vi "Autonomous Independent.vi"() -> ()   [LabVIEW 2015]
doc: "This VI is called when autonomous begins, and will automatically be terminated when autonomous ends. You can carry out timed or sensor driven robot movement independently without needing to return to the caller."
uses:
  Auto States.ctl
  <vilib>/Rock Robotics/WPI/Utilities/WPI_GetSetVariantRefNum.vi
  <vilib>/Rock Robotics/Network Tables/NT Write Numeric Array.vi
  <vilib>/Rock Robotics/Network Tables/NT Read Boolean.vi
  Robot Global Data.vi
  <vilib>/Rock Robotics/Network Tables/NT Read String.vi
  Sensors.vi
panel:
  out "x >= y?":bool
  out "Enum":T1
  out "Complete":bool=TRUE
  out "Crossed":bool
  # "Be sure to right-click and choose Data Operations>>Make Current Value default if you want to save the array values with the VI"
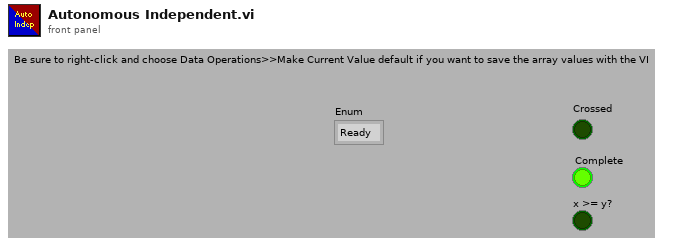
[diagram p1: front panel]
types:
  T1 = typedef "Auto States.ctl" = enum16{"Ready", "Drive to Obstacle", "Cross the Obstacle", "Pause before proceeding", "Position robot for shooting", "Complete"}
  T2 = typedef "WPI_JoystickDevRef.ctl" = cluster{"Device":T3}
  T3 = typedef "WPI_JoystickDeviceEnum.ctl" = enum16{"USB 0", "USB 1", "USB 2", "USB 3", "USB 4", "USB 5"}
  T4 = cluster{"Rotational Value":dbl, "Translational  Value":dbl}
  T5 = typedef "WPI_DigitalInputDevRef.ctl" = cluster{"DevStatus":errorcluster, "DIO Channel":T6}
  T6 = typedef "FPGA_DIOChannel.ctl" = enum8{"DIO 0", "DIO 1", "DIO 2", "DIO 3", "DIO 4", "DIO 5", "DIO 6", "DIO 7", "DIO 8", "DIO 9", "DIO MXP 0", "DIO MXP 1", "DIO MXP 2", "DIO MXP 3", "DIO MXP 4", "DIO MXP 5", "DIO MXP 6", "DIO MXP 7", "DIO MXP 8", "DIO MXP 9", "DIO MXP 10", "DIO MXP 11", "DIO MXP 12", "DIO MXP 13", "DIO MXP 14", "DIO MXP 15", "Invalid"}
  T7 = cluster{"Translational speed":dbl, "Rotational speed":dbl}
  T8 = cluster{"Rotational Velocity Deployed":dbl, "Translational Velocity Deployed":dbl}
  T9 = typedef "WPI_MotorControlDeviceRef.ctl" = cluster{"DeviceStatus":errorcluster, "Type":T10, "PWM":cluster{"PWM Channel":T11, "DeadBand":T12}, "CAN":cluster{"Device Number":u8, "Control Mode":T13, "Semaphore":T14, "Max Vout":dbl, "TalonSRX Control Mode":T15}, "Invert":bool}
  T10 = typedef "WPI_MotorControlType.ctl" = enum16{"PWM", "CAN", "CANTalonSRX"}
  T11 = typedef "FPGA_DIOPWMChannel.ctl" = enum8{"PWM 0", "PWM 1", "PWM 2", "PWM 3", "PWM 4", "PWM 5", "PWM 6", "PWM 7", "PWM 8", "PWM 9", "PWM MXP 0", "PWM MXP 1", "PWM MXP 2", "PWM MXP 3", "PWM MXP 4", "PWM MXP 5", "PWM MXP 6", "PWM MXP 7", "PWM MXP 8", "PWM MXP 9", "Invalid"}
  T12 = typedef "WPI_PWMDeadband.ctl" = cluster{"Name":string, "maxPositivePwm":i32, "minPositivePwm":i32, "centerPwm":i32, "maxNegativePwm":i32, "minNegativePwm":i32, "angularRange":u16}
  T13 = typedef "WPI_CANJaguar_ControlMode.ctl" = enum8{"Percent VBus", "Current", "Speed", "Position", "Voltage"}
  T14 = typedef "Semaphore RefNum" = refnum<k1>
  T15 = typedef "WPI_CANTalonSRX_APIControlMode.ctl" = enum8{"Percent VBus", "Speed", "Position", "Slave", "Unchanged / Invalid", "Voltage Compensation", "Current", "Motion Profile"}
  T16 = typedef "WPI_RobotDriveDevRef.ctl" = cluster{"DevStatus":errorcluster, "Motors[]":T9[], "Square Inputs":bool, "Max Output":dbl}
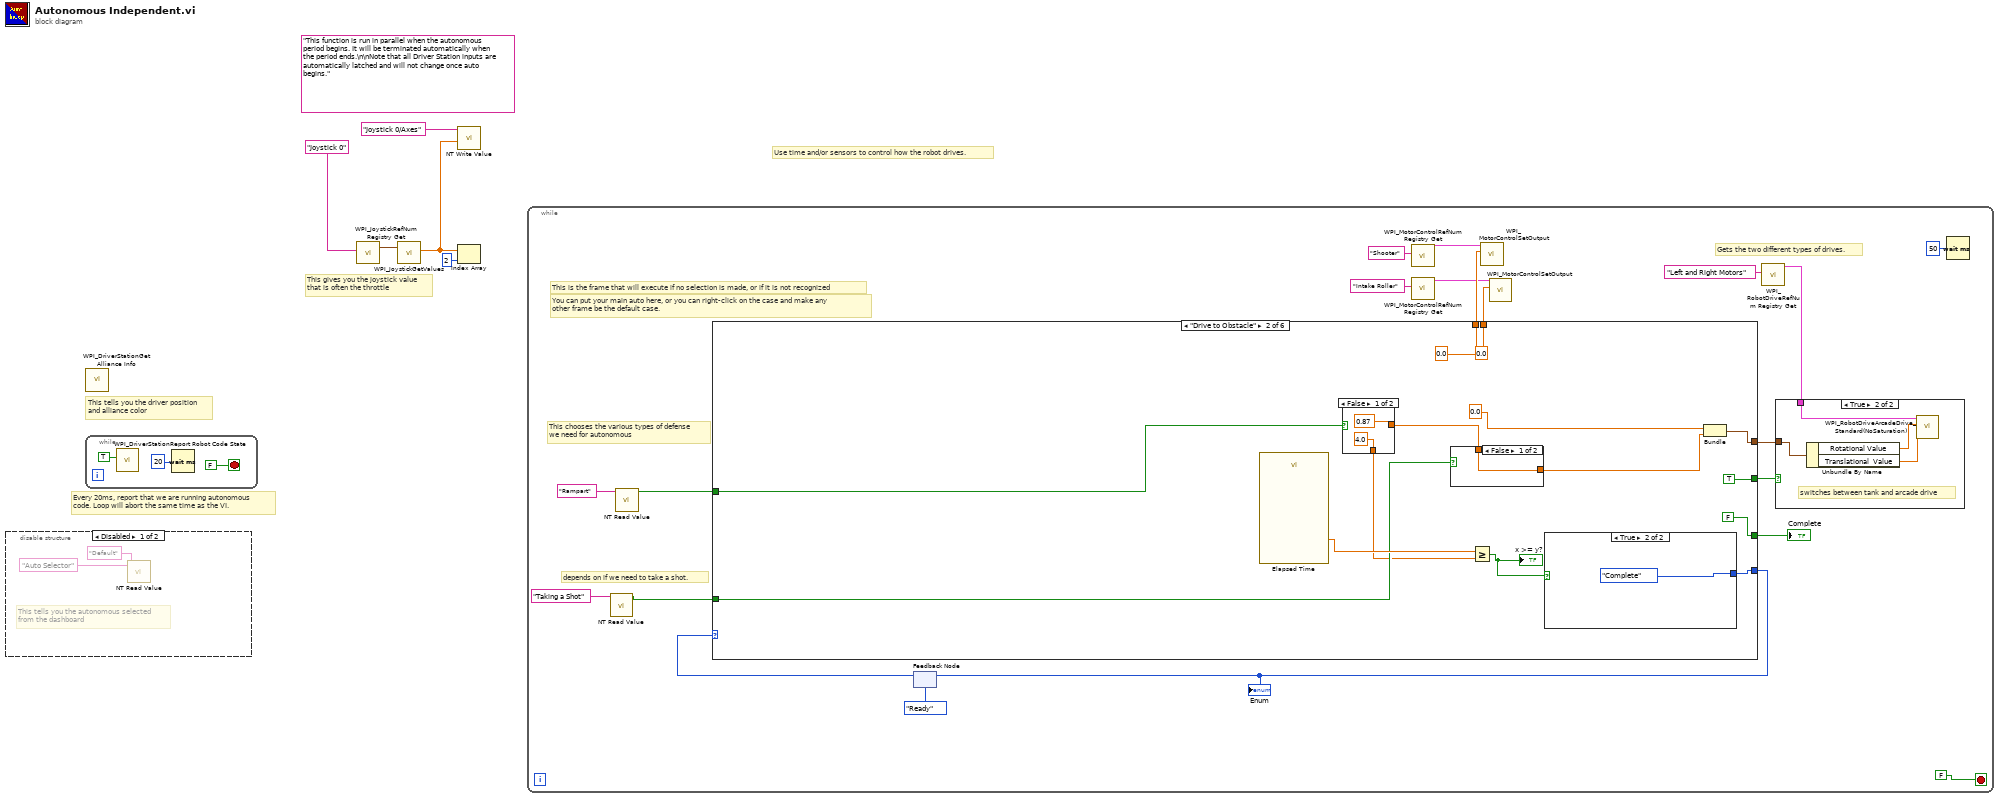
[diagram p0: block diagram]
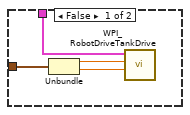
[diagram p2: hidden frame]
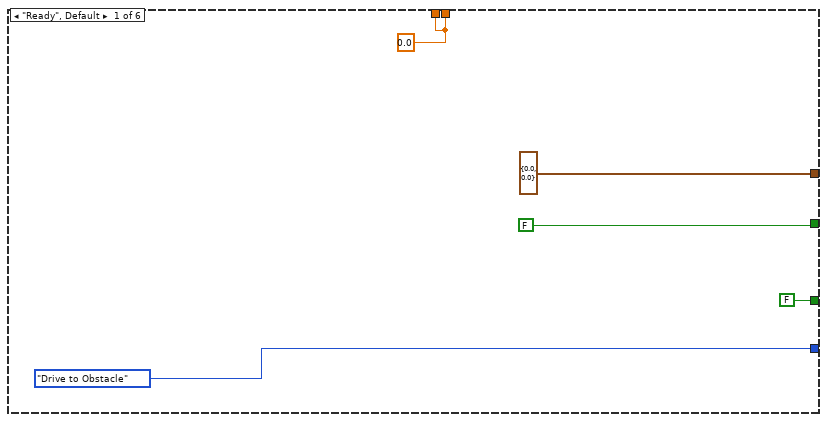
[diagram p3: hidden frame]
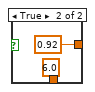
[diagram p4: hidden frame]
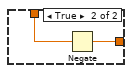
[diagram p5: hidden frame]
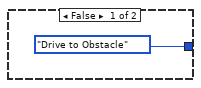
[diagram p6: hidden frame]
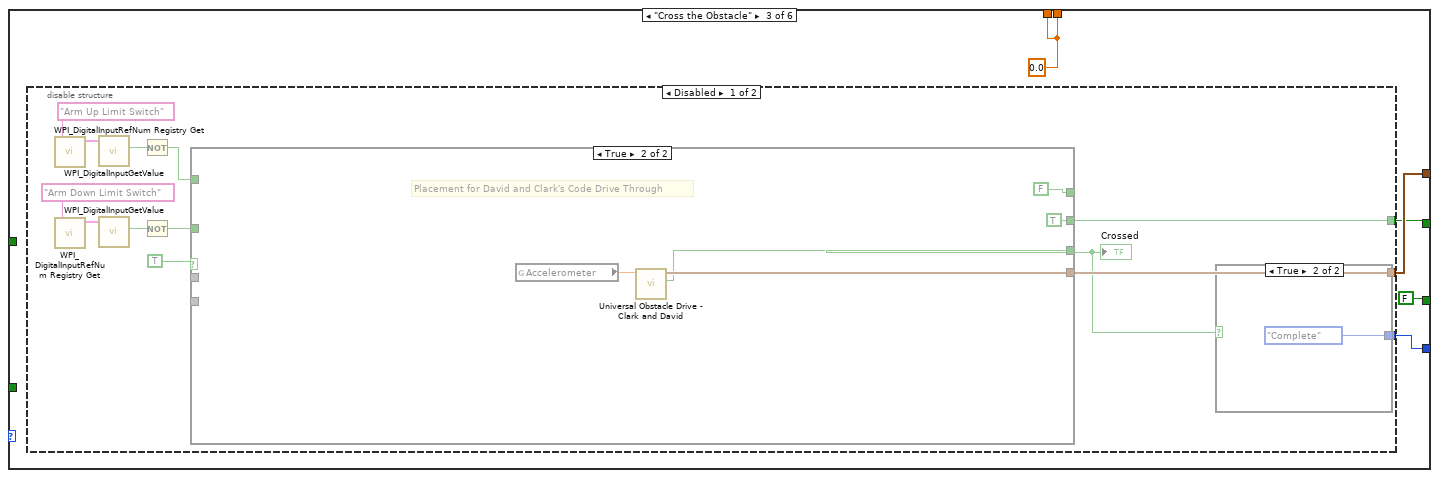
[diagram p7: hidden frame]
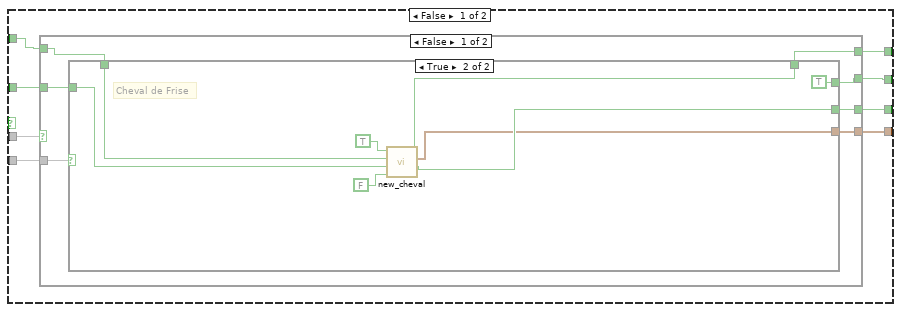
[diagram p8: hidden frame]
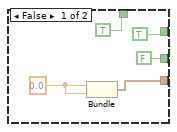
[diagram p9: hidden frame]
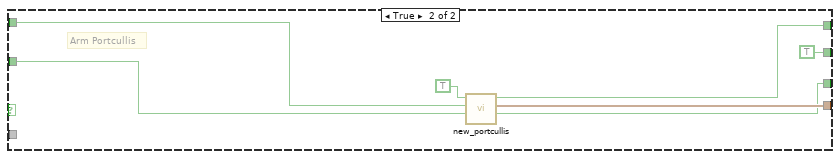
[diagram p10: hidden frame]
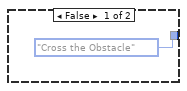
[diagram p11: hidden frame]
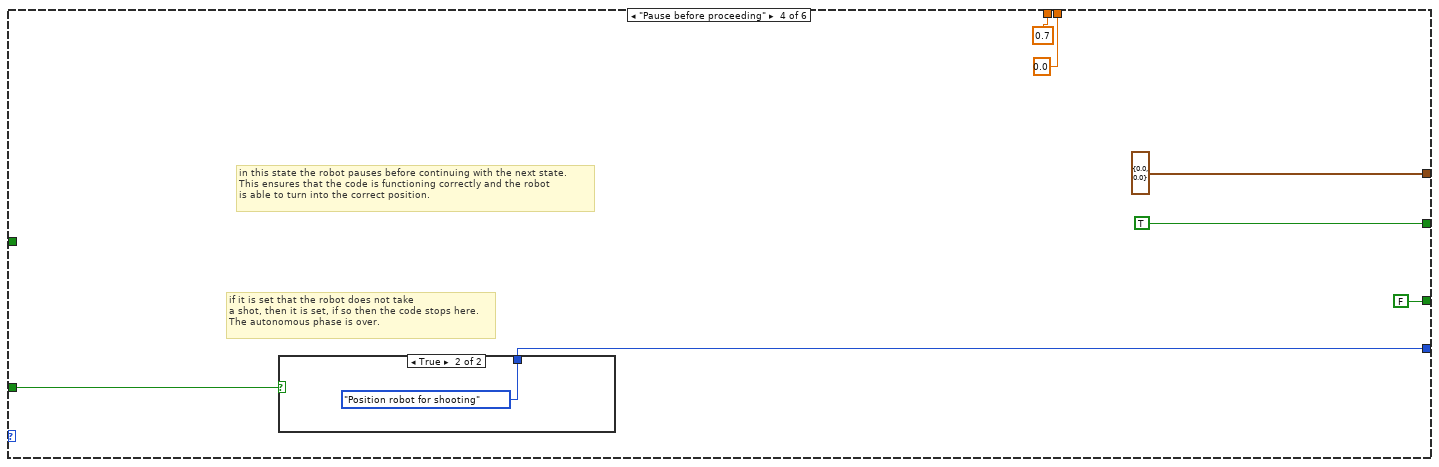
[diagram p13: hidden frame]
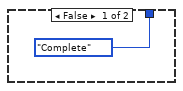
[diagram p14: hidden frame]
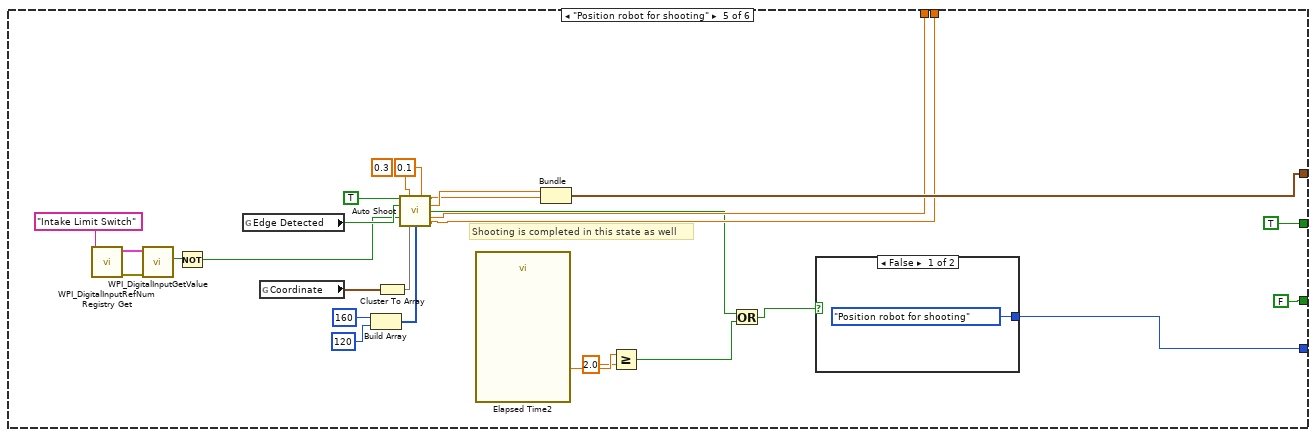
[diagram p15: hidden frame]
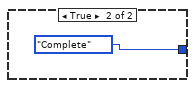
[diagram p16: hidden frame]
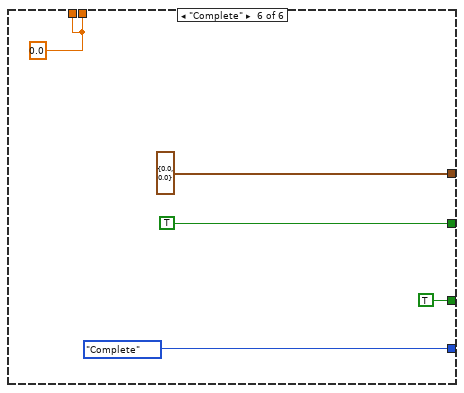
[diagram p17: hidden frame]
diagram:
  (unwired) "This function is run in parallel when the autonomous period begins. It will be terminated automatically when the period ends.\n\nNote that all Driver Station inputs are automatically latched and will not change once auto begins."
  # "Every 20ms, report that we are running autonomous\ncode. Loop will abort the same time as the VI."
  # "This gives you the joystick value\nthat is often the throttle"
  # "Use time and/or sensors to control how the robot drives."
  # "This tells you the driver position\nand alliance color"
  n1 = disable-structure shown="Disabled" {
    frame Disabled {
      # "This tells you the autonomous selected\nfrom the dashboard"
      n2 = call-poly <vilib>:"NT Read Value.vi"("Default Value"="Default", "Name"="Auto Selector") -> ("String"=w7:string)  [unwired: 8 in, 1 out]
    }
    frame Enabled {
    }
  }
  n3 = while {
    stop <- FALSE stop-if-true
    n4 = call <vilib>:"WPI_DriverStationReport Robot Code State.vi"("Autonomous"=TRUE) -> ()  [unwired: 10 in, 1 out]
    n5 = Wait (ms)(milliseconds to wait=u32 20) -> ()  [unwired: 1 out]
  }
  n6 = call <vilib>:"WPI_DriverStationGet Alliance Info.vi"() -> ()  [unwired: 12 out]
  n7 = call <vilib>:"WPI_JoystickRefNum Registry Get.vi"("refnum name"="Joystick 0") -> ("JoystickDevRef"=w4:T2)  [unwired: 1 in, 9 out]
  n8 = call <vilib>:"WPI_JoystickGetValues.vi"("JoystickDevRef"=w4) -> ("Axes"=w2:dbl[])  [unwired: 6 in, 4 out]
  n9 = call-poly <vilib>:"NT Write Value.vi"("Numeric Array"=w2, "Name"="Joystick 0/Axes") -> ()  [unwired: 9 in, 1 out]
  n10 = Index Array(array=w2, index=2) -> ()  [unwired: 1 out]
  n11 = while {
    stop <- FALSE stop-if-true
    # "depends on if we need to take a shot."
    # "Gets the two different types of drives."
    # "This chooses the various types of defense\nwe need for autonomous"
    # "You can put your main auto here, or you can right-click on the case and make any\nother frame be the default case."
    # "This is the frame that will execute if no selection is made, or if it is not recognized"
    n12 = call-poly <vilib>:"NT Read Value.vi"("Name"="Taking a Shot") -> ("Boolean"=w15:bool)  [unwired: 9 in, 1 out]
    n13 = call-poly <vilib>:"NT Read Value.vi"("Name"="Rampart") -> ("Boolean"=w12:bool)  [unwired: 9 in, 1 out]
    n14 = feedback #1(Auto_States."Ready") -> (w23:T1)
    n15 = case shown="\"Drive to Obstacle\"" w23 {
      tunnel: [Auto_States."Drive to Obstacle" w55 w71 w133 w162 Auto_States."Complete"] -> w22
      tunnel: [FALSE TRUE w70 TRUE ("Arcada Drive?") TRUE TRUE ("Arcada Drive?")] -> w30
      tunnel: [T4 {"Rotational Value"=0.0, "Translational  Value"=0.0} ("Aracade Drive") w57 w72 T4 {"Rotational Value"=0.0, "Translational  Value"=0.0} ("Aracade Drive") w159 T4 {"Rotational Value"=0.0, "Translational  Value"=0.0} ("Aracade Drive")] -> w29
      tunnel: w15 -> [_ w49 _ w134 _ _]
      tunnel: [FALSE FALSE FALSE FALSE FALSE TRUE] -> w27
      tunnel: [w40 0.0 w68 0.7 ("Shooter") w151 w165] -> w19
      tunnel: [w40 0.0 w68 0.0 w150 w165] -> w17
      tunnel: w12 -> [_ w45 _ _ _ _]
      frame "Ready", Default {
        w40 = 0.0
      }
      frame "Drive to Obstacle" {
        n16 = call "Elapsed Time"() -> ("Elapsed Time (s)"=w54:dbl)  [unwired: 12 in, 7 out]
        n17 = case shown="False" w45 {
          tunnel: [0.87 0.92 ("Desired Angle")] -> w48
          tunnel: [4.0 6.0 ("y")] -> w46
          frame False {
          }
          frame True {
          }
        }
        n18 = case shown="False" w49 {
          tunnel: w48 -> [w63 w65]
          tunnel: [w63 w64] -> w47
          frame False {
          }
          frame True {
            n19 = Negate(x=w65) -> (-x=w64:dbl)
          }
        }
        n20 = Greater Or Equal?(x=w54, y=w46) -> (x >= y?=w50:bool)
        "x >= y?" <- w50
        n21 = case shown="True" w50 {
          tunnel: [Auto_States."Drive to Obstacle" Auto_States."Complete"] -> w55
          frame False {
          }
          frame True {
          }
        }
        n22 = Bundle("Speed"=0.0, "Desired Angle"=w47) -> (w57:cluster{"Speed":dbl, "Desired Angle":dbl})  [unwired: 1 in]
      }
      frame "Cross the Obstacle" {
        w68 = 0.0
        n23 = disable-structure shown="Disabled" {
          disable-tunnel: [w85 _] -> w72
          disable-tunnel: [w83 _] -> w71
          disable-tunnel: [w82 _] -> w70
          frame Disabled {
            n24 = call <vilib>:"WPI_DigitalInputRefNum Registry Get.vi"("refnum name"="Arm Up Limit Switch") -> ("DigitalInputDevRef"=w81:T5)  [unwired: 9 in, 1 out]
            n25 = call <vilib>:"WPI_DigitalInputRefNum Registry Get.vi"("refnum name"="Arm Down Limit Switch") -> ("DigitalInputDevRef"=w76:T5)  [unwired: 9 in, 1 out]
            n26 = call <vilib>:"WPI_DigitalInputGetValue.vi"("DigitalInputDevRef"=w81) -> ("Value"=w79:bool)  [unwired: 8 in, 2 out]
            n27 = call <vilib>:"WPI_DigitalInputGetValue.vi"("DigitalInputDevRef"=w76) -> ("Value"=w78:bool)  [unwired: 8 in, 2 out]
            n28 = Not(x=w79) -> (.not. x?=w75:bool)
            n29 = Not(x=w78) -> (.not. x?=w74:bool)
            n30 = case shown="True" TRUE {
              tunnel: _ -> [w93 _]
              tunnel: _ -> [w92 _]
              tunnel: [w90 w123] -> w84
              tunnel: [w91 w124] -> w85
              tunnel: [w89 TRUE] -> w82
              tunnel: [w88 FALSE] -> _
              tunnel: w75 -> [w87 _]
              tunnel: w74 -> [w86 _]
              frame False {
                n31 = case shown="False" w93 {
                  tunnel: w92 -> [w100 _]
                  tunnel: [w99 w119] -> w91
                  tunnel: [w98 w117] -> w90
                  tunnel: [w97 TRUE] -> w89
                  tunnel: [w96 w118] -> w88
                  tunnel: w87 -> [w95 w116]
                  tunnel: w86 -> [w94 w115]
                  frame False {
                    n32 = case shown="True" w100 {
                      tunnel: [w103 w111] -> w99
                      tunnel: [FALSE w112] -> w98
                      tunnel: [TRUE TRUE] -> w97
                      tunnel: [TRUE w110] -> w96
                      tunnel: w95 -> [_ w108]
                      tunnel: w94 -> [_ w107]
                      frame False {
                        w104 = 0.0
                        n33 = Bundle(w104, w104) -> (w103:cluster{dbl, dbl})  [unwired: 1 in]
                      }
                      frame True {
                        # "Cheval de Frise"
                        n34 = call "new_cheval.vi"("Abort"=FALSE, "Arm Down"=w107, "Arm Up"=w108, "Start Cheval de Frise"=TRUE) -> ("Done"=w112:bool, "Arcade Drive"=w111:cluster{"x":dbl, "y":dbl}, "Arm Solenoid"=w110:bool)  [unwired: 5 in]
                      }
                    }
                  }
                  frame True {
                    # "Arm Portcullis"
                    n35 = call "new_portcullis.vi"("Arm Down"=w115, "Arm Up"=w116, "Start Portcullis"=TRUE) -> ("Done"=w117:bool, "Arcade Drive"=w119:cluster{"x":dbl, "y":dbl}, "Arm Solenoid"=w118:bool)  [unwired: 6 in]
                  }
                }
              }
              frame True {
                # "Placement for David and Clark's Code Drive Through"
                n36 = global read "Sensors.vi" "Accelerometer"() -> (w125:dbl)
                n37 = call "Universal Obstacle Drive - Clark and David.vi"("Accelerometer"=w125) -> ("Complete"=w123:bool, "Arcade Drive"=w124:T7)  [unwired: 9 in]
              }
            }
            "Crossed" <- w84
            n38 = case shown="True" w84 {
              tunnel: [Auto_States."Cross the Obstacle" Auto_States."Complete"] -> w83
              frame False {
              }
              frame True {
              }
            }
          }
          frame Enabled {
          }
        }
      }
      frame "Pause before proceeding" {
        # "if it is set that the robot does not take\na shot, then it is set, if so then the code stops here.\nThe autonomous phase is over."
        # "in this state the robot pauses before continuing with the next state. \nThis ensures that the code is functioning correctly and the robot\nis able to turn into the correct position."
        n39 = case shown="True" w134 {
          tunnel: [Auto_States."Complete" Auto_States."Position robot for shooting"] -> w133
          frame False {
          }
          frame True {
          }
        }
      }
      frame "Position robot for shooting" {
        w147 = 0.1 ("Rotational Velocity")
        (unwired) 0.3 ("Linear Velocity")
        # "Shooting is completed in this state as well"
        n40 = call <vilib>:"WPI_DigitalInputRefNum Registry Get.vi"("refnum name"="Intake Limit Switch") -> ("error out"=w155:errorcluster, "DigitalInputDevRef"=w156:T5)  [unwired: 9 in]
        n41 = call <vilib>:"WPI_DigitalInputGetValue.vi"("error in (no error)"=w155, "DigitalInputDevRef"=w156) -> ("Value"=w158:bool)  [unwired: 7 in, 2 out]
        n42 = Not(x=w158) -> (.not. x?=w144:bool)
        n43 = global read "Robot Global Data.vi" "Edge Detected"() -> (w145:bool)
        n44 = global read "Robot Global Data.vi" "Coordinate"() -> (w154:cluster{"X":dbl, "Y":dbl})
        n45 = Build Array(160, 120) -> (w142:i32[])
        n46 = Cluster To Array(cluster=w154) -> (array=w143:dbl[])
        n47 = call "Auto Shoot.vi"("Finished Crossing"=TRUE, "Linear Velocity"=w147, "Rotational Velocity"=w147, "Edge Detected"=w145, "Ball In"=w144, "Max Coordinate"=w143, "Image Size"=w142) -> ("Translational Velocity Deployed"=w148:dbl, "Rotational Velocity Deployed"=w149:dbl, "Done"=w138:bool, "Shooter"=w151:dbl, "Intake"=w150:dbl)  [unwired: 4 in]
        n48 = call "Elapsed Time2"() -> ("Elapsed Time (s)"=w141:dbl)  [unwired: 12 in, 7 out]
        n49 = Bundle("Rotational Velocity Deployed"=w149, "Translational Velocity Deployed"=w148) -> (w159:T8)  [unwired: 1 in]
        n50 = Greater Or Equal?(x=w141, y=2.0) -> (x >= y?=w139:bool)
        n51 = Or(x=w138, y=w139) -> (x .or. y?=w137:bool)
        n52 = case shown="False" w137 {
          tunnel: [Auto_States."Position robot for shooting" Auto_States."Complete"] -> w162
          frame False {
          }
          frame True {
          }
        }
      }
      frame "Complete" {
        w165 = 0.0
      }
    }
    "Complete" <- w27
    "Enum" <- w22
    n53 = feedback-in #1(w22) -> ()
    n54 = call <vilib>:"WPI_MotorControlRefNum Registry Get.vi"("refnum name"="Shooter") -> ("MotorControlDevRef"=w18:T9)  [unwired: 9 in, 1 out]
    n55 = call <vilib>:"WPI_MotorControlRefNum Registry Get.vi"("refnum name"="Intake Roller") -> ("MotorControlDevRef"=w16:T9)  [unwired: 9 in, 1 out]
    n56 = call <vilib>:"WPI_MotorControlSetOutput.vi"("Output"=w19, "MotorControlDevRef"=w18) -> ()  [unwired: 7 in, 3 out]
    n57 = call <vilib>:"WPI_MotorControlSetOutput.vi"("Output"=w17, "MotorControlDevRef"=w16) -> ()  [unwired: 7 in, 3 out]
    n58 = call <vilib>:"WPI_RobotDriveRefNum Registry Get.vi"("refnum name"="Left and Right Motors") -> ("RobotDriveDevRef"=w28:T16)  [unwired: 9 in, 1 out]
    n59 = case shown="True" w30 {
      tunnel: w28 -> [w32 w39]
      tunnel: w29 -> [w33 w36]
      frame False {
        n60 = Unbundle(w33) -> ("Rotational Value"=w35:dbl, "Translational  Value"=w34:dbl)
        n61 = call <vilib>:"WPI_RobotDriveTankDrive.vi"("Right axis value"=w34, "Left axis value"=w35, "RobotDriveDevRef"=w32) -> ()  [unwired: 6 in, 3 out]
      }
      frame True {
        # "switches between tank and arcade drive"
        n62 = Unbundle By Name(w36) -> ("Rotational Value"=w38:dbl, "Translational  Value"=w37:dbl)
        n63 = call <vilib>:"WPI_RobotDriveArcadeDrive_Standard(NoSaturation).vi"("Y axis value"=w37, "X axis value"=w38, "RobotDriveDevRef"=w39) -> ()  [unwired: 1 in, 8 out]
      }
    }
    n64 = Wait (ms)(milliseconds to wait=u32 50) -> ()  [unwired: 1 out]
  }
